vi "GetMusicDevices.vi"(0 "reference in":refnum<class "Room.lvclass">, 5 "Error In":errorcluster) -> (14 "reference out":refnum<class "Room.lvclass">, 16 "MusicDevices":refnum<class "MusicDevice.lvclass">[](array[class]), 19 "Error Out":errorcluster)   [LabVIEW 2024, in "Room.lvclass"]
uses:
  Room.lvclass
  Room.lvclass/Room.ctl
  Devices/MusicDevice_class/MusicDevice.lvclass
panel:
  # "Connector Pane"
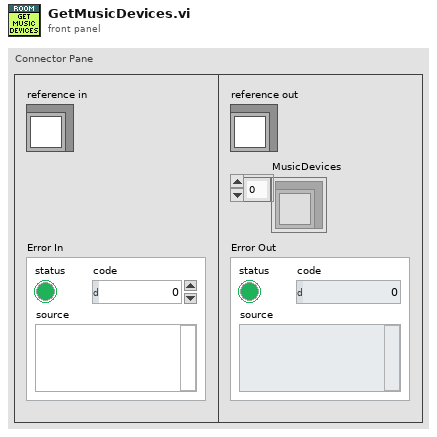
[diagram p1: front panel]
types:
  T1 = typedef "Room.lvclass/ObjectAttributes.ctl" = cluster{"Lights":refnum<class "Light.lvclass">[], "ACs":refnum<class "Air Conditioner.lvclass">[], "Securities":refnum<class "Security.lvclass">[], "MusicDevices":refnum<class "MusicDevice.lvclass">[]}
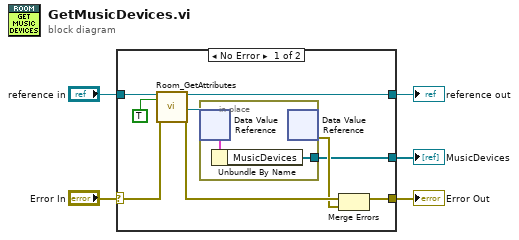
[diagram p0: block diagram]
diagram:
  n1 = case shown="No Error" "Error In" {
    selector: "Error In" -> [w14 w18]
    tunnel: [w12 w18] -> w4
    tunnel: [w9 w17] -> w2
    tunnel: "reference in" -> [w10 w17]
    tunnel: [w6 _] -> w1
    frame No Error {
      n2 = call "Room_GetAttributes.vi"("reference in"=w10, "OnlyGetDvrReference(False)"=TRUE, "Error In"=w14) -> ("reference out"=w9:refnum<class "Room.lvclass">, "DataRef"=w8:refnum<data-value>, "Error Out"=w13:errorcluster)  [unwired: 13 in, 1 out]
      n3 = in-place {
        in-place-border: [w16] -> w6
        n4 = in-place-dvr #1(w8) -> (w15:T1)  [unwired: 1 out]
        n5 = Unbundle By Name(w15) -> ("MusicDevices"=w16:refnum<class "MusicDevice.lvclass">[])
        n6 = in-place-dvr #1() -> (w11:errorcluster)  [unwired: 1 in, 1 out]
      }
      n7 = Merge Errors(w13, w11) -> (w12:errorcluster)
    }
    frame Error {
    }
  }
  "Error Out" <- w4
  "reference out" <- w2
  "MusicDevices" <- w1
